vi "getAllLvPid.vi"(8 "error in (no error)":errorcluster) -> (0 "error out":errorcluster, 3 "PIDs":string[](array[string]))   [LabVIEW 2017, in "BuildWorker Interface.lvlib" / "BuildWorker Controller.lvclass"]
uses:
  BuildWorker Controller.lvclass
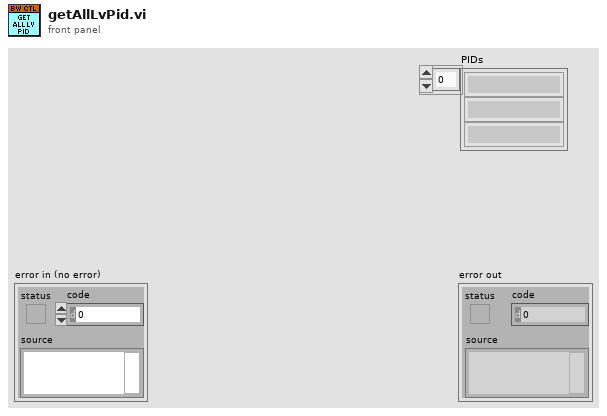
[diagram p1: front panel]
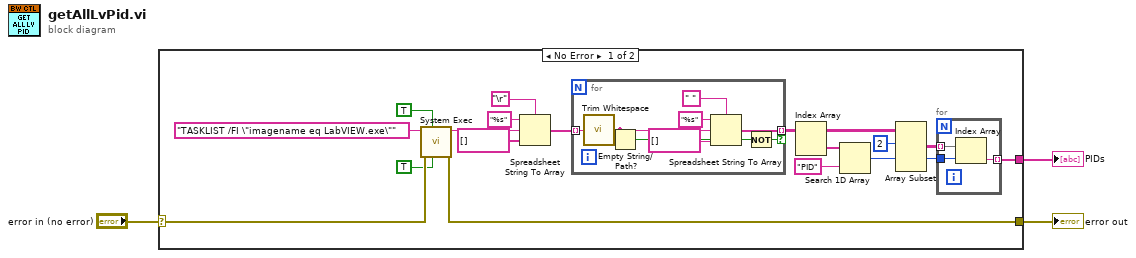
[diagram p0: block diagram]
diagram:
  n1 = case shown="No Error" "error in (no error)" {
    selector: "error in (no error)" -> [w19 w32]
    tunnel: [w18 w32] -> w2
    tunnel: [w4 _] -> w1
    frame No Error {
      n2 = call <vilib>:"System Exec.vi"("run minimized? (F)"=TRUE, "wait until completion? (T)"=TRUE, "error in (no error)"=w19, "command line"="TASKLIST /FI \"imagename eq LabVIEW.exe\"") -> ("error out"=w18:errorcluster, "standard output"=w15:string)  [unwired: 4 in, 2 out]
      n3 = Spreadsheet String To Array(delimiter (Tab)="\r", format string="%s", spreadsheet string=w15, array type (2D Dbl)=string[] []) -> (array=w12:string[])
      n4 = for {
        tunnel: w12 -> [w28] mode=indexing
        tunnel: [w29] -> w8 mode=indexing if=w25
        n5 = call <vilib>:"Trim Whitespace.vi"("string"=w28) -> ("trimmed string"=w24:string)  [unwired: 1 in]
        n6 = Empty String/Path?(string/path=w24) -> (empty?=w27:bool)
        n7 = Spreadsheet String To Array(delimiter (Tab)=" ", format string="%s", spreadsheet string=w24, array type (2D Dbl)=string[] []) -> (array=w29:string[])
        n8 = Not(x=w27) -> (.not. x?=w25:bool)
      }
      n9 = Index Array(array=w8) -> (element=w10:string[])  [unwired: 2 in]
      n10 = Search 1D Array(1D array=w10, element="PID") -> (index of element=w5:i32)  [unwired: 1 in]
      n11 = Array Subset(array=w8, index (row)=2 ("index")) -> (w6:string[][])  [unwired: 3 in]
      n12 = for {
        tunnel: w6 -> [w23] mode=indexing
        tunnel: w5 -> [w22]
        tunnel: [w21] -> w4 mode=indexing
        n13 = Index Array(array=w23, index=w22) -> (element=w21:string)
      }
    }
    frame Error {
    }
  }
  "error out" <- w2
  "PIDs" <- w1
